vi "Create SQL Update Set Clause.vi"(8 "WHERE Clause":string, 9 "Data Types":enum16{"String", "Number", "Date-Time"}[](array[ring])=[enum."String", enum."String", enum."String", enum."String", enum."String", enum."String", enum."Number", enum."Number", enum."Date-Time", enum."String", enum."Number", enum."Number", enum."String", enum."Number", enum."Number", enum."Date-Time", enum."Date-Time", enum."String"], 10 "Column Header Strings[]":string[](array[string]), 11 "New Data":string[](array[string])) -> (3 "SQL Statement":string)   [LabVIEW 2009]
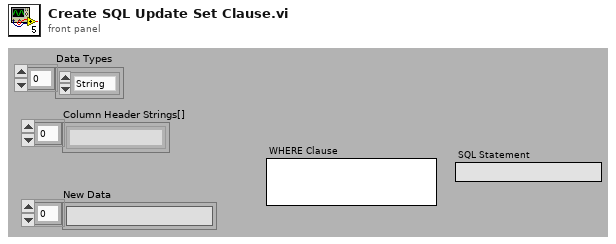
[diagram p1: front panel]
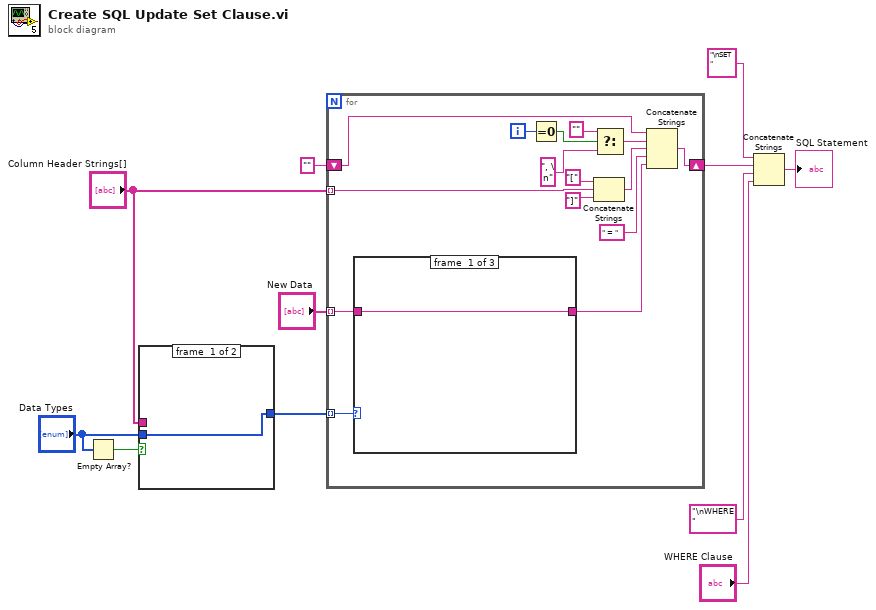
[diagram p0: block diagram]
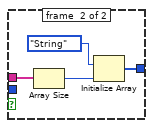
[diagram p2: hidden frame]
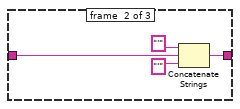
[diagram p3: hidden frame]
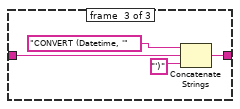
[diagram p4: hidden frame]
diagram:
  n1 = Empty Array?(array="Data Types") -> (empty?=w4:bool)
  n2 = case shown="False" w4 {
    tunnel: "Data Types" -> [w12 _]
    tunnel: [w12 w13] -> w1
    tunnel: "Column Header Strings[]" -> [_ w16]
    frame #0 {
    }
    frame #1 {
      n3 = Array Size(array=w16) -> (size(s)=w15:i32)
      n4 = Initialize Array(enum16{"String", "Number", "Date-Time"}."String", w15) -> (w13:enum16{"String", "Number", "Date-Time"}[])
    }
  }
  n5 = for {
    tunnel: "New Data" -> [w31] mode=indexing
    shift-right: [w28] -> w10
    shift-left: "" -> [w18]
    tunnel: "Column Header Strings[]" -> [w26] mode=indexing
    tunnel: w1 -> [w27] mode=indexing
    i -> [w22]
    n6 = case shown="\"Date-Time\"" w27 {
      tunnel: w31 -> [w32 w34 w38]
      tunnel: [w32 w33 w37] -> w30
      frame #0 {
      }
      frame #1 {
        n7 = Concatenate Strings("'" ("string"), w34, "'" ("string")) -> (w33:string)
      }
      frame #2 {
        n8 = Concatenate Strings("CONVERT (Datetime, '" ("string"), w38, "')" ("string")) -> (w37:string)
      }
    }
    n9 = Equal To 0?(x=w22) -> (x = 0?=w21:bool)
    n10 = Concatenate Strings("[" ("string"), w26, "]" ("string")) -> (w23:string)
    n11 = Select(t="", s=w21, f=", \n" ("string")) -> (s? t:f=w17:string)
    n12 = Concatenate Strings(w18, w17, w23, " = " ("string"), w30) -> (w28:string)
  }
  n13 = Concatenate Strings("\nSET " ("string"), w10, "\nWHERE " ("string"), "WHERE Clause") -> (→"SQL Statement":string)
